vi "Receive Voltage.vi"(8 "error in (no error)":errorcluster, 10 "Receive Voltage":waveform(dbl)[](array[waveform]), 11 "APG in":refnum<class "APG.lvclass">) -> (0 "error out":errorcluster, 3 "APG out":refnum<class "APG.lvclass">)   [LabVIEW 2021, in "APG.lvclass"]
uses:
  APG.lvclass
  APG.lvclass/APG.ctl
  <vilib>/NathanCo/Analog-Tasks/Analog Input/Analog Input/Analog Input/Analog Input.lvclass
  <vilib>/Analysis/NI_AALBase.lvlib
  <vilib>/Analysis/baseanly.llb/Mean (DBL).vi
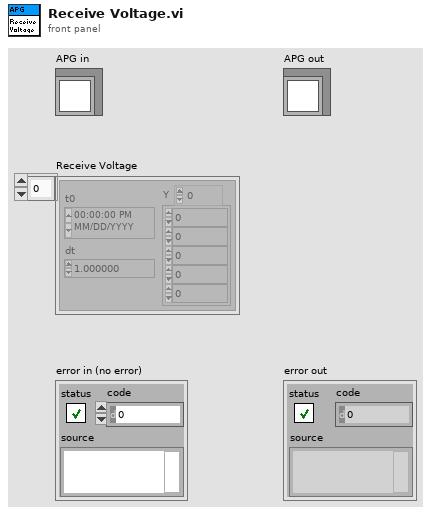
[diagram p1: front panel]
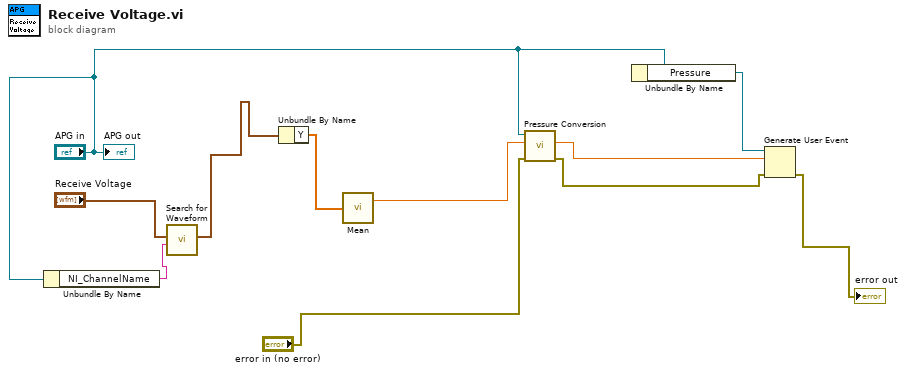
[diagram p0: block diagram]
diagram:
  n1 = Unbundle By Name("APG in") -> ("NI_ChannelName"=w1:string)
  n2 = call <vilib>:"Search for Waveform.vi"("NI_ChannelName"=w1, "Waveforms"="Receive Voltage") -> ("Waveform"=w7:waveform(dbl))  [unwired: 8 in, 1 out]
  n3 = Unbundle By Name(w7) -> ("Y"=w6:dbl[])
  n4 = call-poly <vilib>:"Mean.vi"("X"=w6) -> ("mean"=w5:dbl)  [unwired: 1 out]
  n5 = call "Pressure Conversion.vi"("error in (no error)"="error in (no error)", "Voltage"=w5, "APG in"="APG in") -> ("error out"=w9:errorcluster, "Pressure"=w10:dbl)  [unwired: 7 in]
  n6 = Unbundle By Name("APG in") -> ("Pressure"=w11:refnum<user-event>)
  n7 = Generate User Event(user event=w11, event data cluster=w10, error in=w9) -> (error out=→"error out":errorcluster)  [unwired: 1 in, 1 out]
  "APG out" <- "APG in"
